vi "Remove Element.vi"(8 "error in (no error)":errorcluster, 10 "node Ref":refnum<data-value>, 11 "Priority Queue in":refnum<class "NI_Robotics_Priority Queue.lvclass">) -> (0 "error out":errorcluster, 3 "Priority Queue out":refnum<class "NI_Robotics_Priority Queue.lvclass">)   [LabVIEW 2017, in "NI_Robotics_Priority Queue.lvclass"]
uses:
  <vilib>/robotics/Navigation/shared/Priority Queue/NI_Robotics_Priority Queue.lvclass
  <vilib>/robotics/Navigation/shared/MapNode/AbstractMapNode/NI_Robotics_AbstractMapNode.lvclass
  <vilib>/robotics/Navigation/shared/Priority Queue/NI_Robotics_Priority Queue.lvclass/NI_Robotics_Priority Queue.ctl
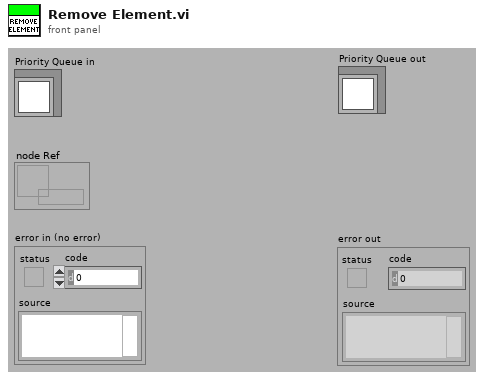
[diagram p1: front panel]
types:
  T1 = typedef "NI_Robotics_Priority Queue.lvclass/Open List Element.ctl" = cluster{"f":dbl, "g":dbl, "node Ref":refnum<data-value>}
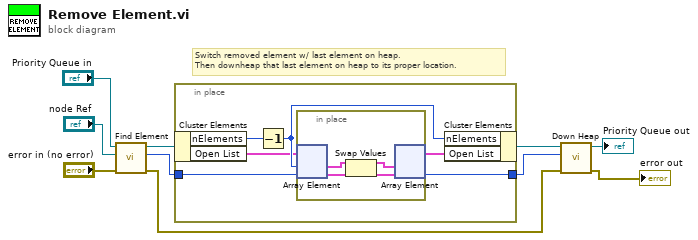
[diagram p0: block diagram]
diagram:
  # "Switch removed element w/ last element on heap.\nThen downheap that last element on heap to its proper location."
  n1 = call <vilib>:"Find Element.vi"("error in (no error)"="error in (no error)", "node Ref"="node Ref", "Priority Queue in"="Priority Queue in") -> ("error out"=w1:errorcluster, "Numeric"=w6:i32, "Priority Queue out"=w7:refnum<class "NI_Robotics_Priority Queue.lvclass">)  [unwired: 6 in]
  n2 = in-place {
    in-place-border: w6 -> [w14]
    in-place-border: [w11] -> w3
    n3 = in-place-cluster #1(w7) -> ("nElements"=w16:i32, "Open List"=w13:T1[])
    n4 = Decrement(x=w16) -> (x-1=w15:i32)
    n5 = in-place {
      n6 = in-place-array #2(w13, w15, w14) -> (w20:T1, w19:T1)
      n7 = Swap Values(12:w20, 14:w19) -> (1:w18:T1, 3:w17:T1)  [unwired: 1 in]
      n8 = in-place-array #2(w18, w17) -> (w12:T1[], w11:i32)  [unwired: 1 out]
    }
    n9 = in-place-cluster #1("nElements"=w15, "Open List"=w12) -> (w5:refnum<class "NI_Robotics_Priority Queue.lvclass">)
  }
  n10 = call <vilib>:"Down Heap.vi"("error in (no error)"=w1, "index"=w3, "Astar Open List in"=w5) -> ("error out"=→"error out":errorcluster, "Astar Open List out"=→"Priority Queue out":refnum<class "NI_Robotics_Priority Queue.lvclass">)  [unwired: 7 in]
